vi "Hex to Packets.vi"(0 "AOL_Globals":T1={"Imaging Protocol"=enum."AOL Z-Stack", "Number of POI"=0, "Number of Miniscans"=0, "Number of Trials"=0, "Number of Cycles "=0, "# Averaged Frames"=0, "Laser power (%)"=0, "Pockels"=0.0, "Acquisition Length (sec)"=0.0, "Fill time (us)"=0.0, "POI Dwell time (us)"=0.0, "Miniscan Dwell time per pixel (us)"=0.0, "PMT 1"=0.0, "PMT 2"=0.0, "Back Apperture"=0.0, "Frame Size"=0, "Center Frequency"=0.0, "Field of View"=0.0, "DwellTime (us)"=0.0, "Wavelength (nm)"=0.0, "Zoom"=0.0, "AOL Z"=0.0, "AOL Mode"=enum."Raster", "GridXY"=0.0, "GridZ"=0.0, "TriggerPeriod (sec)"=0.0, "Number of Pixels in Miniscan"=0, "Experiment folder path"=path "", "X centre"=0.0, "Y centre"=0.0, "Angle (degrees)"=0.0, "Plane Mode"=0, "Threshold"=[], "Regenerate Chirps"=FALSE, "Rectangle ROI length (pixels)"=0, "Rectangle ROI height (pixels)"=0, "AOD fill"=0, "Samples Wait after Trigger"=0, "StartUp Delay"=0, "Slip Cycle"=163840, "Add Cycle"=FALSE} {"Plane Mode" items=["XY Plane"]; "Frame Size" items=["100X100"=100, "128X128"=128, "200X200"=200, "256X256"=256, "512X512"=512, "1024x1024"=1024, "2048x2048"=2048]; "Back Apperture" format="%#.6g"; "Pockels" format="%#.6g"; "PMT 2" format="%#.6g"; "PMT 1" format="%#.6g"; "Angle (degrees)" format="%#.6g"; "POI Dwell time (us)" format="%#.6g"}, 2 "MAC Address":string, 5 "Hex Array":string[](array[string]), 7 "Nx":i32, 9 "Ny":i32) -> (4 "Packets":string[](array[string]), 10 "Interrupted":bool)   [LabVIEW 2013]
uses:
  Typedefs/Controls/AOL_Globals.ctl
  Typedefs/Imaging Protocols enum.ctl
  Typedefs/Frame Size.ctl
  Typedefs/AOL modes.ctl
  Typedefs/Plane Mode.ctl
  Global Variables/General Globals.vi
panel:
  out "resized  Hex array":string[][](array[string])
  out "resized array size":i32[](array[numeric])
  out "num records":i32
  out "command_load_pts":string
  out "string":string
  out "strart index":i32
  out "end index":i32
  # "RE-ENTRANT"
  # "SUB-ROUTINE"
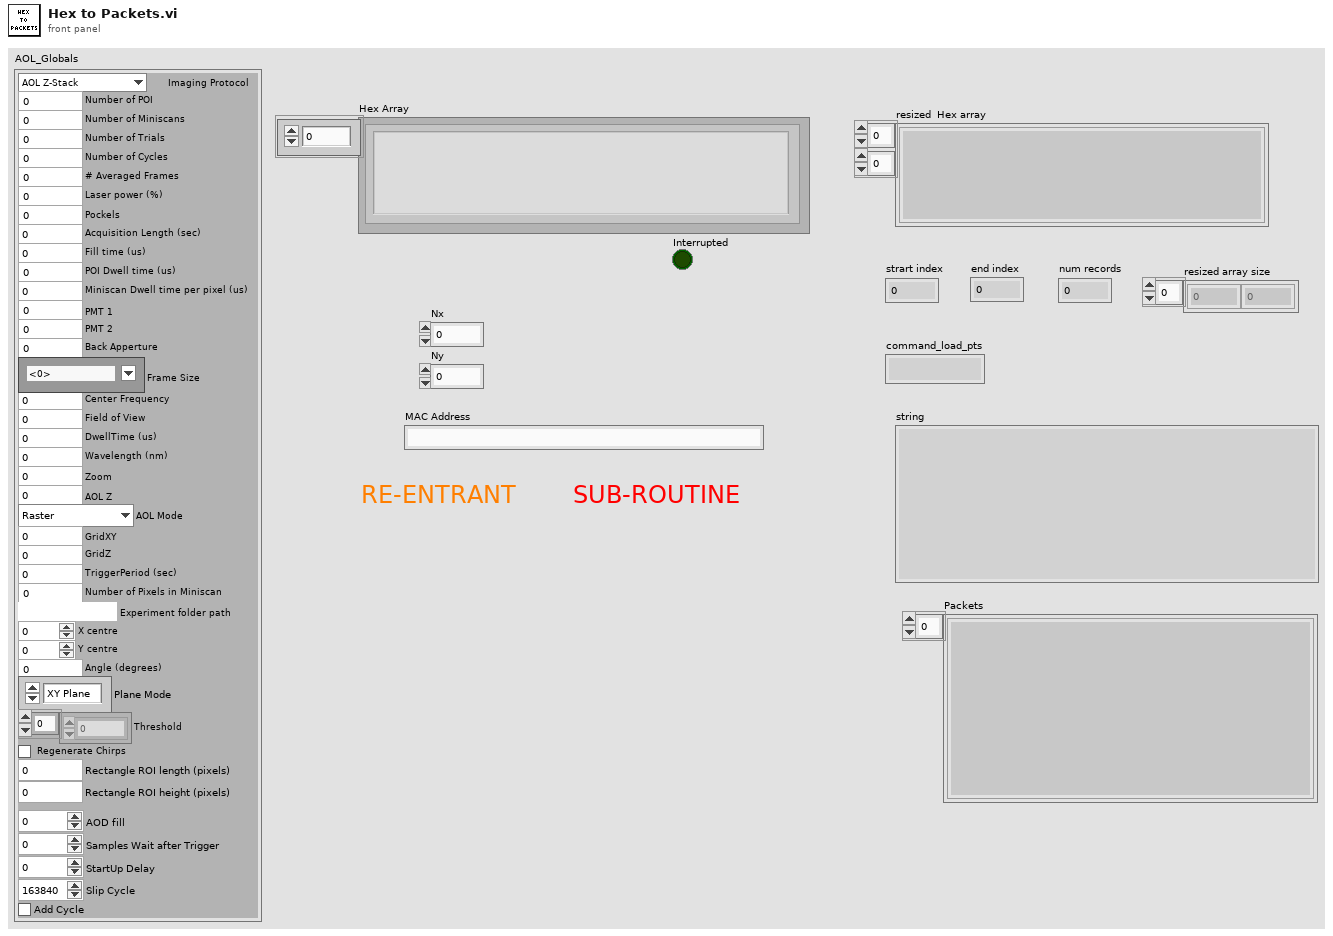
[diagram p1: front panel]
types:
  T1 = typedef "AOL_Globals.ctl" = cluster{"Imaging Protocol":T2, "Number of POI":u16, "Number of Miniscans":u16, "Number of Trials":u16, "Number of Cycles ":u64, "# Averaged Frames":u16, "Laser power (%)":u8, "Pockels":dbl, "Acquisition Length (sec)":dbl, "Fill time (us)":dbl, "POI Dwell time (us)":dbl, "Miniscan Dwell time per pixel (us)":dbl, "PMT 1":dbl, "PMT 2":dbl, "Back Apperture":dbl, "Frame Size":T3, "Center Frequency":dbl, "Field of View":dbl, "DwellTime (us)":dbl, "Wavelength (nm)":dbl, "Zoom":dbl, "AOL Z":dbl, "AOL Mode":T4, "GridXY":dbl, "GridZ":dbl, "TriggerPeriod (sec)":dbl, "Number of Pixels in Miniscan":u16, "Experiment folder path":path, "X centre":dbl, "Y centre":dbl, "Angle (degrees)":dbl, "Plane Mode":T5, "Threshold":u16[], "Regenerate Chirps":bool, "Rectangle ROI length (pixels)":u16, "Rectangle ROI height (pixels)":u16, "AOD fill":u16, "Samples Wait after Trigger":u16, "StartUp Delay":i32, "Slip Cycle":u32, "Add Cycle":bool}
  T2 = typedef "Imaging Protocols enum.ctl" = enum16{"AOL Z-Stack", "Motor Z Stack", "Functional Acquisition", "Single Plane Acquisition", "Volume Acquisition", "Live Imaging", "Live Plane Imaging", "Live Volume Imaging"}
  T3 = typedef "Frame Size.ctl" = u16
  T4 = typedef "AOL modes.ctl" = enum16{"Raster", "Structural", "Pointing", "Mini Scan", "Alignment"}
  T5 = typedef "Plane Mode.ctl" = u16
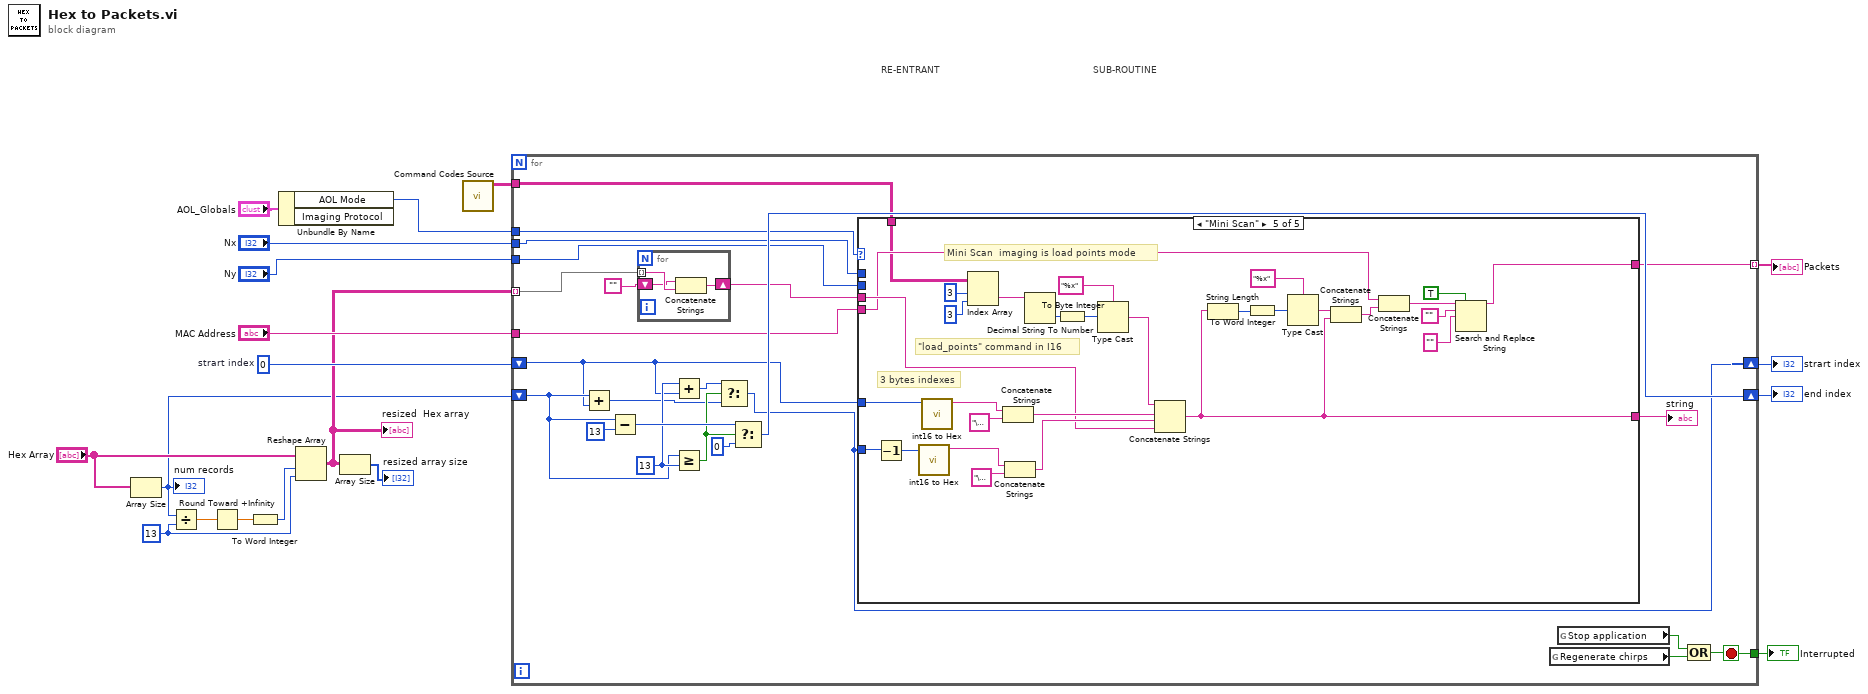
[diagram p0: block diagram]
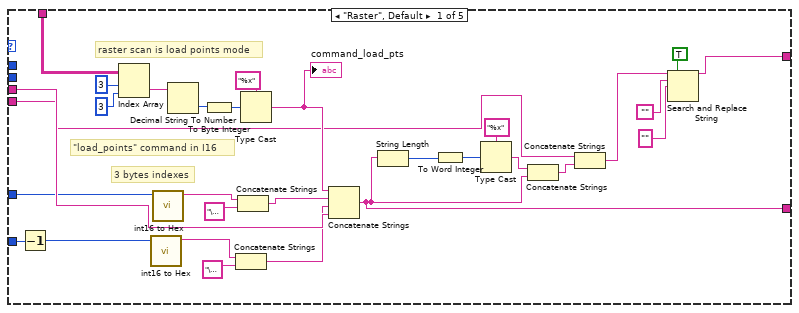
[diagram p2: hidden frame]
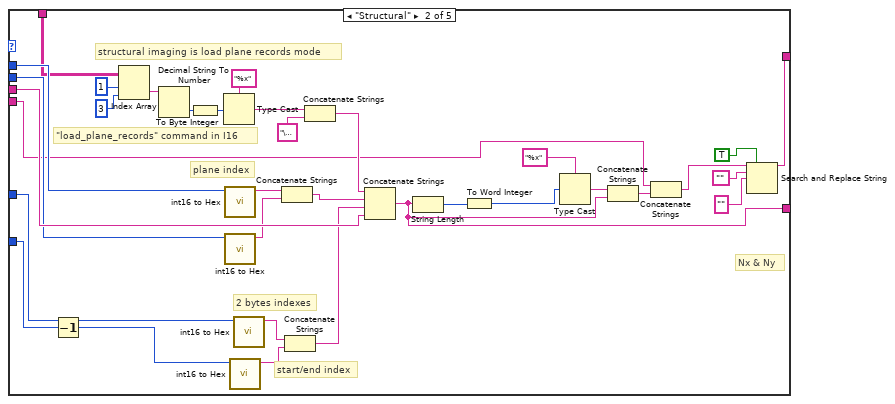
[diagram p3: hidden frame]
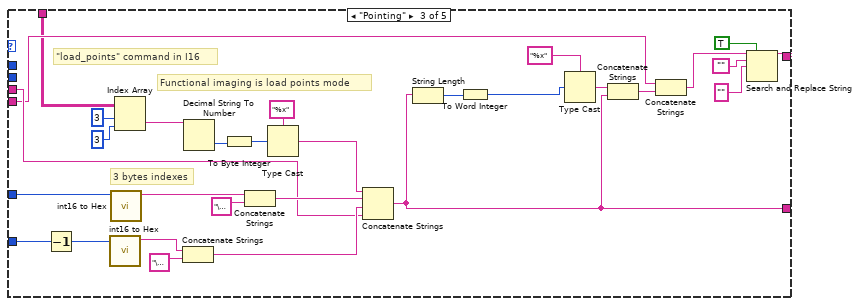
[diagram p4: hidden frame]
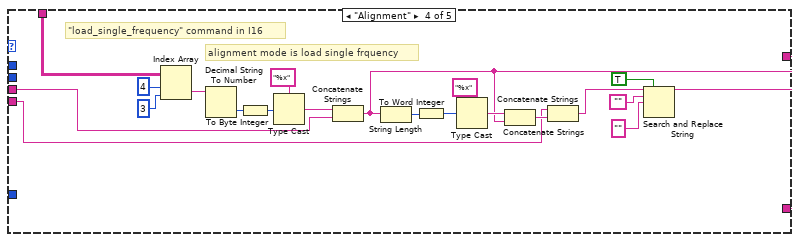
[diagram p5: hidden frame]
diagram:
  w8 = 13 ("y")
  w15 = 0  # strart index
  # "SUB-ROUTINE"
  # "RE-ENTRANT"
  n1 = Array Size(array="Hex Array") -> (size(s)=w3:i32)
  "num records" <- w3
  n2 = Divide(x=w3, y=w8) -> (x/y=w10:dbl)
  n3 = Round Toward +Infinity(x=w10) -> (ceil(x): smallest int >= x=w9:dbl)
  n4 = To Word Integer(number=w9) -> (16bit integer=w5:i16)
  n5 = Unbundle By Name("AOL_Globals") -> ("AOL Mode"=w11:T4)  [unwired: 1 out]
  n6 = Reshape Array("Hex Array", w5, w8) -> (w4:string[][])
  "resized  Hex array" <- w4
  n7 = Array Size(array=w4) -> (size(s)=→"resized array size":i32[])
  n8 = call "Command Codes Source.vi"() -> ("Commands for FPGA"=w1:string[][])  [unwired: 11 in]
  n9 = for {
    shift-right: [w41] -> w14
    shift-left: w3 -> [w36]
    shift-right: [w25] -> w13
    shift-left: w15 -> [w29]
    tunnel: w4 -> [w33] mode=indexing
    tunnel: w11 -> [w32]
    tunnel: [w30] -> w18 mode=indexing
    tunnel: "Nx" -> [w27]
    tunnel: "Ny" -> [w26]
    tunnel: "MAC Address" -> [w24]
    tunnel: w1 -> [w23]
    tunnel: [w21] -> w2
    stop <- w21 stop-if-true
    w37 = 13 ("y")
    n10 = Add(x=w36, y=w29) -> (x+y=w35:i32)
    n11 = Subtract(x=w36, y=13) -> (x-y=w42:i32)
    n12 = for {
      tunnel: w33 -> [w191] mode=indexing
      shift-right: [w190] -> w31
      shift-left: "" -> [w189]
      n13 = Concatenate Strings(w189, w191) -> (w190:string)
    }
    n14 = Add(x=w37, y=w29) -> (x+y=w38:i32)
    n15 = Greater Or Equal?(x=w36, y=w37) -> (x >= y?=w39:bool)
    n16 = Select(t=w38, s=w39, f=w35) -> (s? t:f=w25:i32)
    n17 = Select(t=w42, s=w39, f=0) -> (s? t:f=w41:i32)
    n18 = case shown="\"Mini Scan\"" w32 {
      tunnel: w31 -> [w64 w107 w114 w142 w163]
      tunnel: [w49 w97 w113 w141 w162] -> w30
      tunnel: w29 -> [w57 w82 w115 _ w164]
      tunnel: w25 -> [w51 w81 w111 _ w165]
      tunnel: [w47 w77 w112 w140 w159] -> w28
      tunnel: w27 -> [_ w87 _ _ _]
      tunnel: w26 -> [_ w86 _ _ _]
      tunnel: w24 -> [w44 w75 w109 w139 w161]
      tunnel: w23 -> [w45 w74 w108 w138 w160]
      frame "Raster", Default {
        # "\"load_points\" command in I16"
        # "3 bytes indexes"
        # "raster scan is load points mode"
        n19 = Decrement(x=w51) -> (x-1=w46:i32)
        n20 = Index Array(array=w45, index (row)=3 ("disabled index (row)"), index (col)=3 ("disabled index (col)")) -> (element=w58:string)
        n21 = call "int16 to Hex.vi"("number"=w46) -> ("Hex string"=w53:string)  [unwired: 10 in]
        n22 = call "int16 to Hex.vi"("number"=w57) -> ("Hex string"=w56:string)  [unwired: 10 in]
        n23 = Decimal String To Number(string=w58) -> (number=w60:i32)  [unwired: 2 in, 1 out]
        n24 = To Byte Integer(number=w60) -> (8bit integer=w59:i8)
        n25 = Concatenate Strings(w53, "\u0000" ("string")) -> (w50:string)
        n26 = Concatenate Strings(w56, "\u0000" ("string")) -> (w54:string)
        n27 = Type Cast(type="%x", x=w59) -> (*(type *) &x=w48:string)
        "command_load_pts" <- w48
        n28 = Concatenate Strings(w48, w54, w50, w64) -> (w47:string)
        n29 = String Length(string=w47) -> (length=w70:i32)
        n30 = To Word Integer(number=w70) -> (16bit integer=w65:i16)
        n31 = Type Cast(type="%x", x=w65) -> (*(type *) &x=w72:string)
        n32 = Concatenate Strings(w72, w47) -> (w73:string)
        n33 = Concatenate Strings(w44, w73) -> (w69:string)
        n34 = Search and Replace String(replace all?=TRUE ("replace all? (F)"), input string=w69, search string="", replace string="" ("replace string (\"\")")) -> (result string=w49:string)  [unwired: 4 in, 3 out]
      }
      frame "Structural" {
        # "\"load_plane_records\" command in I16"
        # "start/end index"
        # "2 bytes indexes"
        # "Nx & Ny"
        # "plane index"
        # "structural imaging is load plane records mode"
        n35 = Decrement(x=w81) -> (x-1=w76:i32)
        n36 = Index Array(array=w74, index (row)=1 ("disabled index (row)"), index (col)=3 ("disabled index (col)")) -> (element=w91:string)
        n37 = Decimal String To Number(string=w91) -> (number=w93:i32)  [unwired: 2 in, 1 out]
        n38 = To Byte Integer(number=w93) -> (8bit integer=w92:i8)
        n39 = Type Cast(type="%x", x=w92) -> (*(type *) &x=w90:string)
        n40 = call "int16 to Hex.vi"("number"=w87) -> ("Hex string"=w85:string)  [unwired: 10 in]
        n41 = call "int16 to Hex.vi"("number"=w86) -> ("Hex string"=w84:string)  [unwired: 10 in]
        n42 = call "int16 to Hex.vi"("number"=w76) -> ("Hex string"=w79:string)  [unwired: 10 in]
        n43 = call "int16 to Hex.vi"("number"=w82) -> ("Hex string"=w80:string)  [unwired: 10 in]
        n44 = Concatenate Strings(w85, w84) -> (w83:string)
        n45 = Concatenate Strings(w80, w79) -> (w78:string)
        n46 = Concatenate Strings(w90, "\u0000" ("string")) -> (w88:string)
        n47 = Concatenate Strings(w88, w83, w78, w107) -> (w77:string)
        n48 = String Length(string=w77) -> (length=w103:i32)
        n49 = To Word Integer(number=w103) -> (16bit integer=w98:i16)
        n50 = Type Cast(type="%x", x=w98) -> (*(type *) &x=w105:string)
        n51 = Concatenate Strings(w105, w77) -> (w106:string)
        n52 = Concatenate Strings(w75, w106) -> (w102:string)
        n53 = Search and Replace String(replace all?=TRUE ("replace all? (F)"), input string=w102, search string="", replace string="" ("replace string (\"\")")) -> (result string=w97:string)  [unwired: 4 in, 3 out]
      }
      frame "Pointing" {
        # "\"load_points\" command in I16"
        # "3 bytes indexes"
        # "Functional imaging is load points mode"
        n54 = Decrement(x=w111) -> (x-1=w110:i32)
        n55 = call "int16 to Hex.vi"("number"=w110) -> ("Hex string"=w119:string)  [unwired: 10 in]
        n56 = call "int16 to Hex.vi"("number"=w115) -> ("Hex string"=w122:string)  [unwired: 10 in]
        n57 = Index Array(array=w108, index (row)=3 ("disabled index (row)"), index (col)=3 ("disabled index (col)")) -> (element=w123:string)
        n58 = Concatenate Strings(w119, "\u0000" ("string")) -> (w117:string)
        n59 = Decimal String To Number(string=w123) -> (number=w125:i32)  [unwired: 2 in, 1 out]
        n60 = To Byte Integer(number=w125) -> (8bit integer=w124:i8)
        n61 = Concatenate Strings(w122, "\u0000" ("string")) -> (w120:string)
        n62 = Type Cast(type="%x", x=w124) -> (*(type *) &x=w116:string)
        n63 = Concatenate Strings(w116, w120, w117, w114) -> (w112:string)
        n64 = String Length(string=w112) -> (length=w134:i32)
        n65 = To Word Integer(number=w134) -> (16bit integer=w129:i16)
        n66 = Type Cast(type="%x", x=w129) -> (*(type *) &x=w136:string)
        n67 = Concatenate Strings(w136, w112) -> (w137:string)
        n68 = Concatenate Strings(w109, w137) -> (w133:string)
        n69 = Search and Replace String(replace all?=TRUE ("replace all? (F)"), input string=w133, search string="", replace string="" ("replace string (\"\")")) -> (result string=w113:string)  [unwired: 4 in, 3 out]
      }
      frame "Alignment" {
        # "\"load_single_frequency\" command in I16"
        # "alignment mode is load single frquency"
        n70 = Index Array(array=w138, index (row)=4 ("disabled index (row)"), index (col)=3 ("disabled index (col)")) -> (element=w144:string)
        n71 = Decimal String To Number(string=w144) -> (number=w146:i32)  [unwired: 2 in, 1 out]
        n72 = To Byte Integer(number=w146) -> (8bit integer=w145:i8)
        n73 = Type Cast(type="%x", x=w145) -> (*(type *) &x=w143:string)
        n74 = Concatenate Strings(w143, w142) -> (w140:string)
        n75 = String Length(string=w140) -> (length=w155:i32)
        n76 = To Word Integer(number=w155) -> (16bit integer=w150:i16)
        n77 = Type Cast(type="%x", x=w150) -> (*(type *) &x=w157:string)
        n78 = Concatenate Strings(w157, w140) -> (w158:string)
        n79 = Concatenate Strings(w139, w158) -> (w154:string)
        n80 = Search and Replace String(replace all?=TRUE ("replace all? (F)"), input string=w154, search string="", replace string="" ("replace string (\"\")")) -> (result string=w141:string)  [unwired: 4 in, 3 out]
      }
      frame "Mini Scan" {
        # "\"load_points\" command in I16"
        # "3 bytes indexes"
        # "Mini Scan  imaging is load points mode"
        n81 = Decrement(x=w165) -> (x-1=w166:i32)
        n82 = call "int16 to Hex.vi"("number"=w166) -> ("Hex string"=w170:string)  [unwired: 10 in]
        n83 = call "int16 to Hex.vi"("number"=w164) -> ("Hex string"=w173:string)  [unwired: 10 in]
        n84 = Index Array(array=w160, index (row)=3 ("disabled index (row)"), index (col)=3 ("disabled index (col)")) -> (element=w174:string)
        n85 = Concatenate Strings(w173, "\u0000" ("string")) -> (w171:string)
        n86 = Concatenate Strings(w170, "\u0000" ("string")) -> (w168:string)
        n87 = Decimal String To Number(string=w174) -> (number=w176:i32)  [unwired: 2 in, 1 out]
        n88 = To Byte Integer(number=w176) -> (8bit integer=w175:i8)
        n89 = Type Cast(type="%x", x=w175) -> (*(type *) &x=w167:string)
        n90 = Concatenate Strings(w167, w171, w168, w163) -> (w159:string)
        n91 = String Length(string=w159) -> (length=w185:i32)
        n92 = To Word Integer(number=w185) -> (16bit integer=w180:i16)
        n93 = Type Cast(type="%x", x=w180) -> (*(type *) &x=w187:string)
        n94 = Concatenate Strings(w187, w159) -> (w188:string)
        n95 = Concatenate Strings(w161, w188) -> (w184:string)
        n96 = Search and Replace String(replace all?=TRUE ("replace all? (F)"), input string=w184, search string="", replace string="" ("replace string (\"\")")) -> (result string=w162:string)  [unwired: 4 in, 3 out]
      }
    }
    "string" <- w28
    n97 = global read "General Globals.vi" "Regenerate chirps"() -> (w22:bool)
    n98 = global read "General Globals.vi" "Stop application"() -> (w20:bool)
    n99 = Compound Arithmetic op=OR(w20, w22) -> (w21:bool)
  }
  "Packets" <- w18
  "end index" <- w14
  "strart index" <- w13
  "Interrupted" <- w2
